vi "WriteDebugLine.vi"(10 "Data To Write":string, 11 "Mode":enum16{"Open", "Write Line", "Close"}(ring)) -> ()   [LabVIEW 2014]
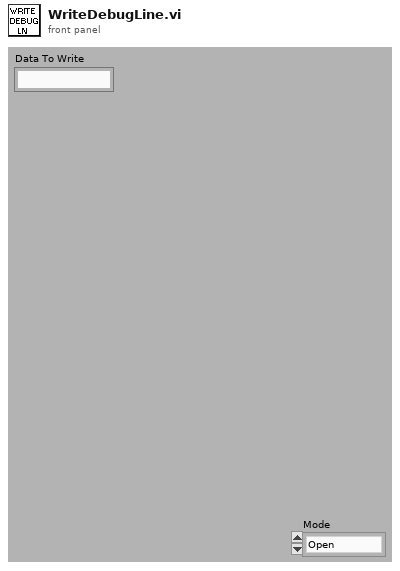
[diagram p1: front panel]
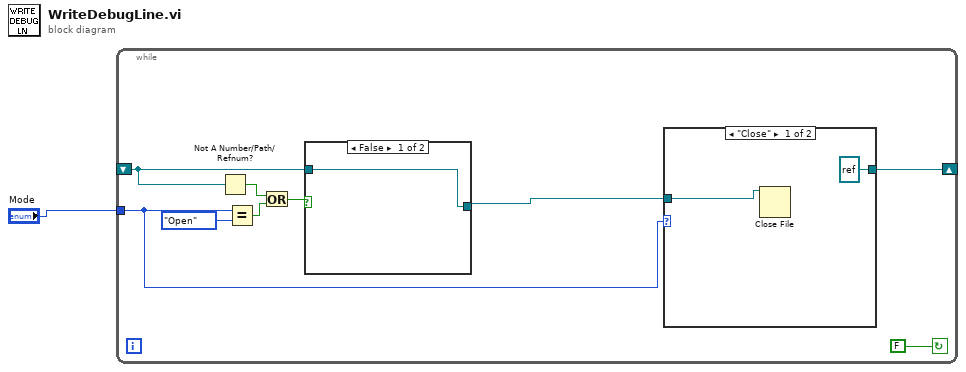
[diagram p0: block diagram]
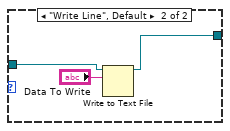
[diagram p2: hidden frame]
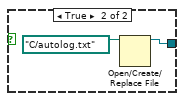
[diagram p3: hidden frame]
diagram:
  n1 = while {
    shift-right: [w4] -> _
    shift-left: _ -> [w3]
    tunnel: "Mode" -> [w6]
    stop <- FALSE continue-if-true
    n2 = Not A Number/Path/Refnum?(number/path/refnum=w3) -> (NaN/Path/Refnum?=w7:bool)
    n3 = Equal?(x=w6, y=enum16{"Open", "Write Line", "Close"}."Open") -> (x = y?=w9:bool)
    n4 = Or(x=w7, y=w9) -> (x .or. y?=w10:bool)
    n5 = case shown="False" w10 {
      tunnel: [w16 w17] -> w5
      tunnel: w3 -> [w16 _]
      frame False {
      }
      frame True {
        n6 = Open/Create/Replace File(file path (use dialog)=path "C:/autolog.txt") -> (refnum out=w17:refnum<file>)  [unwired: 1 in, 6 out]
      }
    }
    n7 = case shown="\"Close\"" w6 {
      tunnel: w5 -> [w12 w14]
      tunnel: [refnum<file> refnum ("refnum out") w13] -> w4
      frame "Close" {
        n8 = Close File(refnum=w12) -> ()  [unwired: 1 in, 2 out]
      }
      frame "Write Line", Default {
        n9 = Write to Text File(file (use dialog)=w14, text="Data To Write") -> (refnum out=w13:refnum<file>)  [unwired: 1 in, 3 out]
      }
    }
  }
